vi "Lian_Lab08_I.vi"() -> ()   [LabVIEW 2020]
uses:
  <vilib>/DAQmx/read.llb/DAQmx Read (Analog 2D DBL NChan NSamp).vi
  <vilib>/DAQmx/create/channels.llb/DAQmx Create Channel (AI-Voltage-Basic).vi
  <vilib>/DAQmx/configure/timing.llb/DAQmx Timing (Sample Clock).vi
  <vilib>/DAQmx/miscellaneous.llb/DAQmx Fill In Error Info.vi
panel:
  out "Waveform Chart":dbl[][](graph)
  in  "number of samples \nper channel":i32=10
  in  "?":bool
  in  "Loop Multiple (ms)":u32
  in  "Rate":dbl=100.0 format="%0.2f"
  in  "Samples per Channel":i32=1000
  in  "Physical Channels":tag="myDAQ1/ai0:1"
  in  "Maximum Voltage":dbl=10.0 format="%0.2f"
  in  "Minimum Voltage":dbl=-10.0 format="%0.2f"
  in  "Input Terminal Config.":i32(ring)=10106 items=["Default"=-1, "RSE"=10083, "NRSE"=10078, "Differential"=10106, "Pseudodifferential"=12529]
  # "Part I. Multiple Analog Inputs"
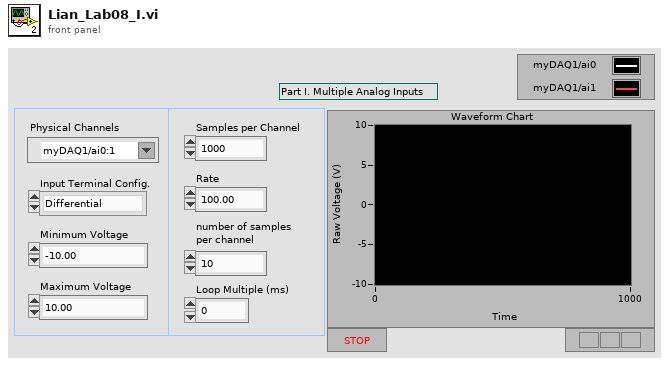
[diagram p1: front panel]
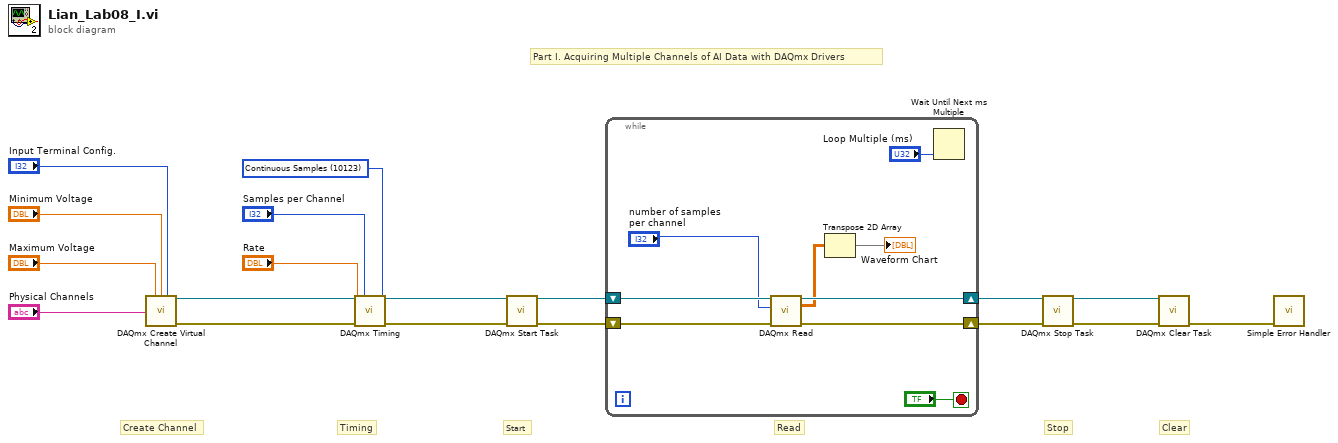
[diagram p0: block diagram]
diagram:
  w1 = 10123 items=["Finite Samples"=10178, "Continuous Samples"=10123, "Hardware Timed Single Point"=12522] ("sample mode")
  # "Part I. Acquiring Multiple Channels of AI Data with DAQmx Drivers"
  # "Clear"
  # "Stop"
  # "Read"
  # "Start"
  # "Timing"
  # "Create Channel"
  n1 = call-poly <vilib>:"DAQmx Create Virtual Channel.vi"("maximum value"="Maximum Voltage", "minimum value"="Minimum Voltage", "input terminal configuration"="Input Terminal Config.", "physical channels"="Physical Channels") -> ("task out"=w7:refnum<k21>, "error out"=w13:errorcluster)  [unwired: 10 in]
  n2 = call-poly <vilib>:"DAQmx Timing.vi"("task/channels in"=w7, "sample mode"=w1, "samples per channel"="Samples per Channel", "rate"="Rate", "error in"=w13) -> ("task out"=w6:refnum<k21>, "error out"=w12:errorcluster)  [unwired: 9 in]
  n3 = call <vilib>:"DAQmx Start Task.vi"("task/channels in"=w6, "error in"=w12) -> ("task out"=w5:refnum<k21>, "error out"=w11:errorcluster)  [unwired: 12 in]
  n4 = while {
    shift-right: [w26] -> w10
    shift-left: w11 -> [w27]
    shift-right: [w24] -> w4
    shift-left: w5 -> [w25]
    stop <- "?" stop-if-true
    n5 = call-poly <vilib>:"DAQmx Read.vi"("task/channels in"=w25, "number of samples per channel"="number of samples \nper channel", "error in"=w27) -> ("task out"=w24:refnum<k21>, "data"=w20:dbl[][], "error out"=w26:errorcluster)  [unwired: 10 in]
    n6 = Transpose 2D Array(2D array=w20) -> (transposed array=→"Waveform Chart":dbl[][])
    n7 = Wait Until Next ms Multiple(millisecond multiple="Loop Multiple (ms)") -> ()  [unwired: 1 out]
  }
  n8 = call <vilib>:"DAQmx Stop Task.vi"("task/channels in"=w4, "error in"=w10) -> ("task out"=w3:refnum<k21>, "error out"=w9:errorcluster)  [unwired: 12 in]
  n9 = call <vilib>:"DAQmx Clear Task.vi"("task in"=w3, "error in"=w9) -> ("error out"=w8:errorcluster)  [unwired: 13 in]
  n10 = call <vilib>:"Simple Error Handler.vi"("error in (no error)"=w8) -> ()  [unwired: 4 in, 5 out]
